vi "E700-Inverter Control.vi"(8 "error in (no error)":errorcluster, 9 "Direction Switch":bool, 10 "ON/OFF - Switch":bool, 11 "Modbus Master in":refnum<class "Modbus Master.lvclass">) -> (0 "error out":errorcluster, 3 "Modbus Master out":refnum<class "Modbus Master.lvclass">)   [LabVIEW 2020]
uses:
  <vilib>/NI/Modbus Library/API/Master/Modbus Master.lvclass
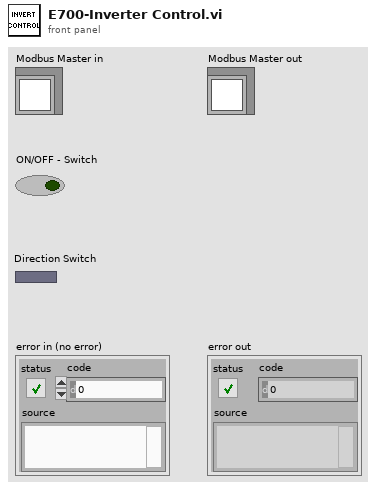
[diagram p1: front panel]
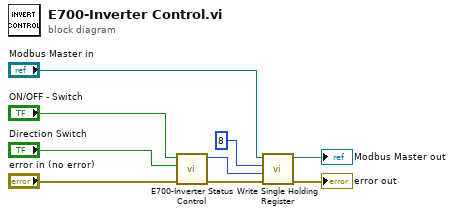
[diagram p0: block diagram]
diagram:
  n1 = call "E700-Inverter Status Control.vi"("error in (no error)"="error in (no error)", "Direction Switch"="Direction Switch", "ON/OFF - Switch"="ON/OFF - Switch") -> ("error out"=w2:errorcluster, "Send Value"=w4:u16)  [unwired: 7 in]
  n2 = call-dynamic "Write Single Holding Register.vi"("error in"=w2, "register to write"=w4, "address"=u16 8, "Modbus master in"="Modbus Master in") -> ("error out"=→"error out":errorcluster, "Modbus master out"=→"Modbus Master out":refnum<class "Modbus Master.lvclass">)  [unwired: 6 in]
